vi "search_for_closest.vi"(9 "search center":dbl, 10 "input array":dbl[](array[numeric]), 11 "start index":i32) -> (3 "closest element":i32)   [LabVIEW 2014]
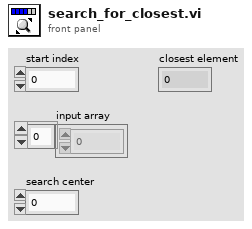
[diagram p1: front panel]
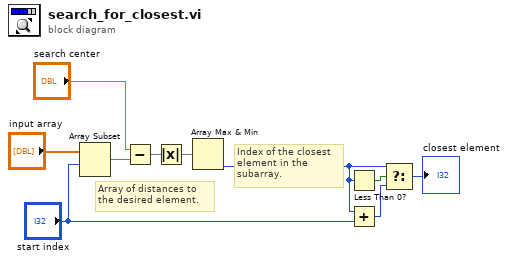
[diagram p0: block diagram]
diagram:
  # "Array of distances to the desired element."
  # "Index of the closest element in the subarray."
  n1 = Array Subset(array="input array", index="start index") -> (w6:dbl[])  [unwired: 1 in]
  n2 = Subtract(x="search center", y=w6) -> (x-y=w1:dbl[])
  n3 = Absolute Value(x=w1) -> (abs(x)=w2:dbl[])
  n4 = Array Max & Min(array=w2) -> (min index (indices)=w4:i32)  [unwired: 3 out]
  n5 = Less Than 0?(x=w4) -> (x < 0?=w3:bool)
  n6 = Add(x=w4, y="start index") -> (x+y=w5:i32)
  n7 = Select(t=w4, s=w3, f=w5) -> (s? t:f=→"closest element":i32)
